vi "Handle setAllData.vi"(8 "error in (no error)":errorcluster, 10 "AllData":variant, 11 "Instrument.Framework-Template in":refnum<class "Instrument.Framework-Template.lvclass">) -> (0 "error out":errorcluster, 3 "Instrument.Framework-Template out":refnum<class "Instrument.Framework-Template.lvclass">)   [LabVIEW 2019, in "Instrument.Framework-Template.lvclass"]
doc: "Override to handle \"getAll\" or \"getAllData\" commands for <b>your</b> Instrument"
uses:
  Instrument.Framework-Template.lvclass
  Instrument.Framework-Template.lvclass/Instrument.Framework-Template.ctl
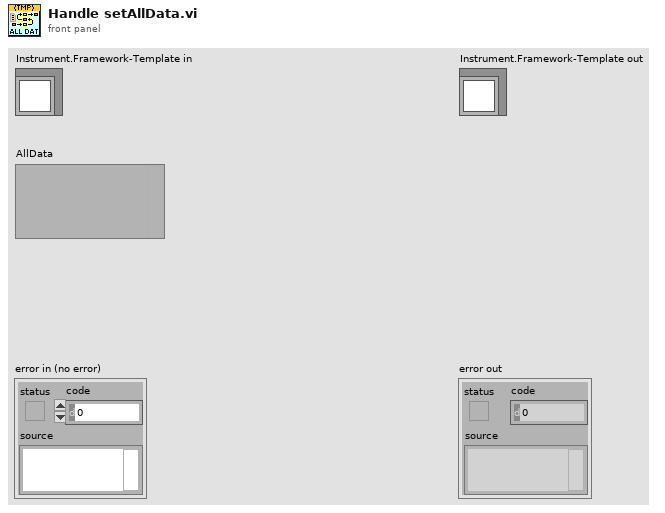
[diagram p1: front panel]
types:
  T1 = typedef "Instrument.Framework-Template.lvclass/Instrument.Framework-Template.getAll--Cluster.ctl" = cluster{"Levy 1":dbl, "Logger SMO":dbl, "SMO Boolean":bool, "SMO String":string}
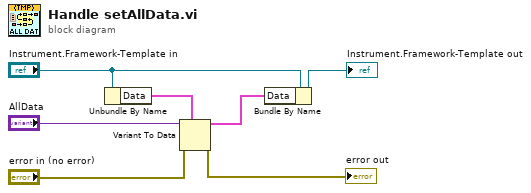
[diagram p0: block diagram]
diagram:
  n1 = Unbundle By Name("Instrument.Framework-Template in") -> ("Data"=w5:T1)
  n2 = Variant To Data(error in="error in (no error)", type=w5, Variant="AllData") -> (data=w3:T1, error out=→"error out":errorcluster)
  n3 = Bundle By Name(cluster="Instrument.Framework-Template in", "Data"=w3) -> (→"Instrument.Framework-Template out":refnum<class "Instrument.Framework-Template.lvclass">)
